vi "SweepIV.vi"(3 "error in (no error)":errorcluster, 4 "StepSize":dbl, 5 "VISA resource name":refnum<visa-resource-name>) -> (0 "error out":errorcluster, 1 "Sweep":sgl[][](array[numeric]), 2 "VISA resource name out":refnum<visa-resource-name>)   [LabVIEW 2012]
uses:
  <instrlib>/Keithley 24XX/Public/Data/Read (Multiple Points).vi
  <vilib>/Utility/file.llb/Write To Spreadsheet File (DBL).vi
  <instrlib>/Keithley 24XX/Keithley 24XX.lvlib
panel:
  in  "Device":string
  out "XY Graph 2":cluster{"Voltage":sgl[], "Current":sgl[]}(graph)
  out "XY Graph":cluster{"Voltage":sgl[], "Current":sgl[]}(graph)
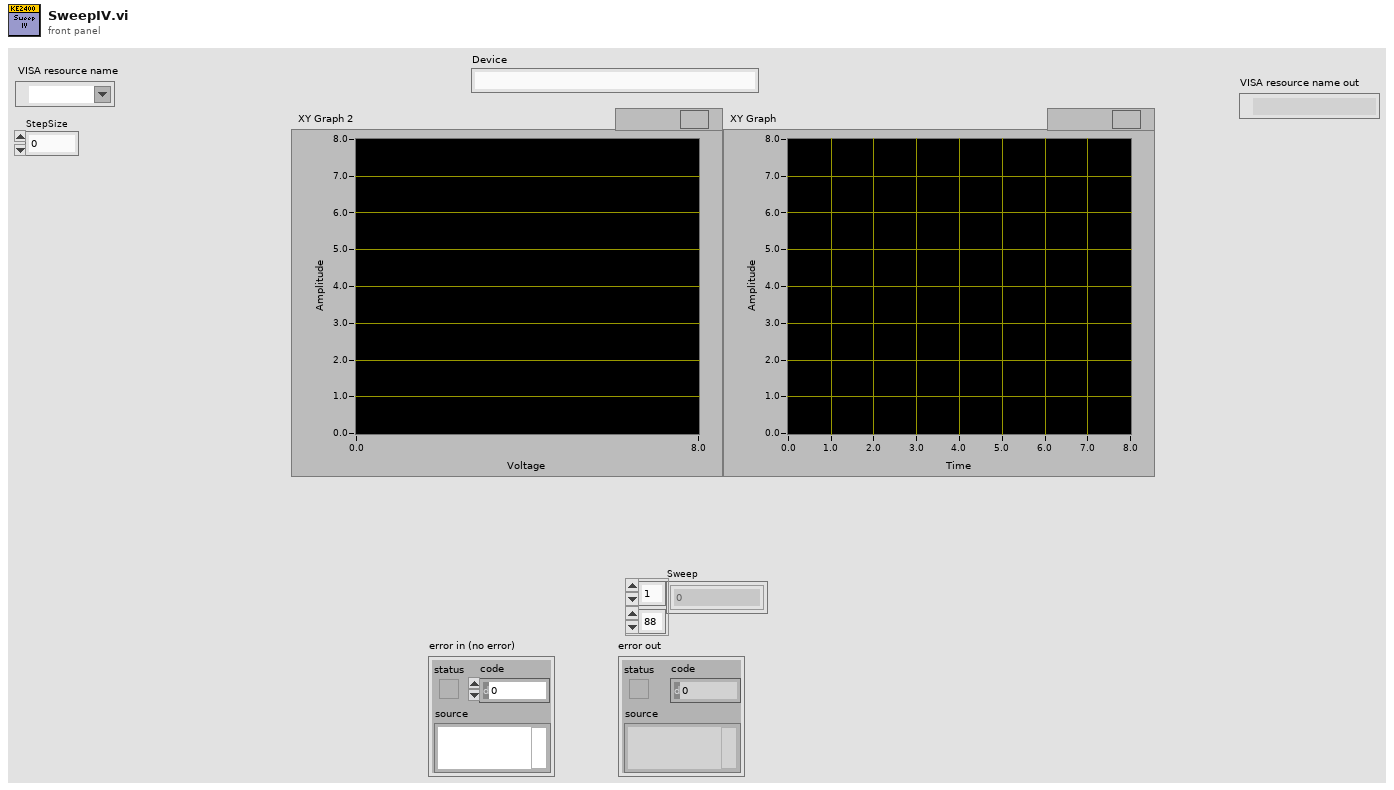
[diagram p1: front panel]
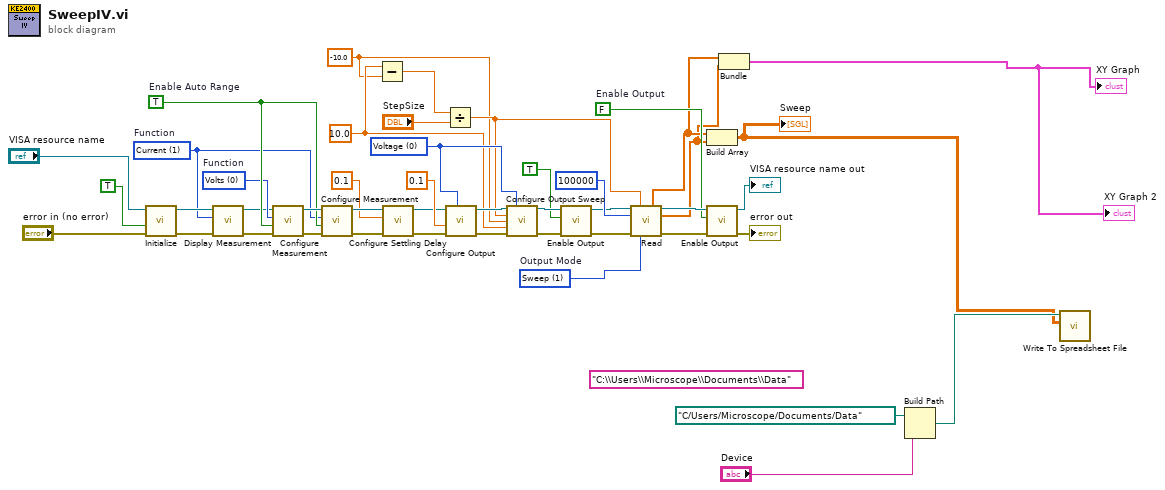
[diagram p0: block diagram]
diagram:
  (unwired) "C:\\Users\\Microscope\\Documents\\Data"
  w23 = 10.0 ("Maximum Amplitude (2)")
  w22 = -10.0 ("Minimum Amplitude (1)")
  w29 = u16 0 items=["Voltage", "Current"] ("Source Mode  (0: Voltage)")
  w31 = TRUE  # Enable Auto Range
  w8 = u16 1 items=["Volts", "Current", "Resistance"]  # Function
  w16 = u16 0 items=["Volts", "Current", "Resistance"]  # Function
  w37 = FALSE  # Enable Output
  w40 = u16 1 items=["Fixed", "Sweep", "List"]  # Output Mode
  n1 = call <instrlib>:"Initialize.vi"("error in (no error)"="error in (no error)", "Reset (True)"=TRUE, "VISA resource name"="VISA resource name") -> ("error out"=w19:errorcluster, "VISA resource name out"=w20:refnum<visa-resource-name>)  [unwired: 7 in]
  n2 = call <instrlib>:"Display Measurement.vi"("error in (no error)"=w19, "Displayed Measurement (0: Voltage)"=w8, "VISA resource name"=w20) -> ("error out"=w15:errorcluster, "VISA resource name out"=w14:refnum<visa-resource-name>)  [unwired: 7 in]
  n3 = call <instrlib>:"Configure Measurement.vi"("error in (no error)"=w15, "Enable Auto Range (T:Enable)"=w31, "Function (0: Volts)"=w16, "VISA resource name"=w14) -> ("error out"=w45:errorcluster, "VISA resource name out"=w44:refnum<visa-resource-name>)  [unwired: 6 in]
  n4 = call <instrlib>:"Configure Measurement.vi"("error in (no error)"=w45, "Enable Auto Range (T:Enable)"=w31, "Function (0: Volts)"=w8, "VISA resource name"=w44) -> ("error out"=w12:errorcluster, "VISA resource name out"=w13:refnum<visa-resource-name>)  [unwired: 6 in]
  n5 = Subtract(x=w23, y=w22) -> (x-y=w26:dbl)
  n6 = call <instrlib>:"Configure Settling Delay.vi"("error in (no error)"=w12, "Manual Settling Delay (0 sec)"=0.1, "VISA resource name"=w13) -> ("error out"=w9:errorcluster, "VISA resource name out"=w10:refnum<visa-resource-name>)  [unwired: 7 in]
  n7 = Divide(x=w26, y="StepSize") -> (x/y=w24:dbl)
  n8 = call <instrlib>:"Configure Output.vi"("Source Mode  (0: Voltage)"=w29, "error in (no error)"=w9, "Compliance  Level (0.1)"=0.1, "VISA resource name"=w10) -> ("error out"=w43:errorcluster, "VISA resource name out"=w42:refnum<visa-resource-name>)  [unwired: 6 in]
  n9 = call <instrlib>:"Configure Output Sweep.vi"("VISA resource name"=w42, "Source Mode  (0: Voltage)"=w29, "Number of Points (5)"=w24, "Minimum Amplitude (1)"=w22, "Maximum Amplitude (2)"=w23, "error in (no error)"=w43) -> ("VISA resource name out"=w34:refnum<visa-resource-name>, "error out"=w33:errorcluster)  [unwired: 8 in]
  n10 = call <instrlib>:"Enable Output.vi"("error in (no error)"=w33, "Enable Output (T: Enable)"=TRUE ("Enable Output"), "VISA resource name"=w34) -> ("error out"=w36:errorcluster, "VISA resource name out"=w35:refnum<visa-resource-name>)  [unwired: 7 in]
  n11 = call-poly <instrlib>:"Read.vi"("VISA resource name"=w35, "Sample Count (1)"=w24, "Timeout (10000 ms)"=100000, "error in (no error)"=w36, "Output Mode (0: Fixed)"=w40) -> ("Voltage"=w7:sgl[], "VISA resource name out"=w38:refnum<visa-resource-name>, "Current"=w6:sgl[], "error out"=w39:errorcluster)  [unwired: 4 in, 3 out]
  n12 = Build Array(w7, w6) -> (w1:sgl[][])
  "Sweep" <- w1
  n13 = call <instrlib>:"Enable Output.vi"("error in (no error)"=w39, "Enable Output (T: Enable)"=w37, "VISA resource name"=w38) -> ("error out"=→"error out":errorcluster, "VISA resource name out"=→"VISA resource name out":refnum<visa-resource-name>)  [unwired: 7 in]
  n14 = Bundle("Voltage"=w7, "Current"=w6) -> (→"XY Graph" →"XY Graph 2":cluster{"Voltage":sgl[], "Current":sgl[]})  [unwired: 1 in]
  n15 = Build Path(base path=path "C:/Users/Microscope/Documents/Data", name or relative path="Device") -> (appended path=w2:path)
  n16 = call-poly <vilib>:"Write To Spreadsheet File.vi"("2D data"=w1, "file path (dialog if empty)"=w2) -> ()  [unwired: 6 in, 1 out]
